vi "Multiply.vi"() -> ()   [LabVIEW 2014]
doc: "Use this template to build a VI to use as a subVI."
uses:
  <vilib>/vision/NI_Vision_Development_Module.lvlib
panel:
  out "Src":T1(plugin-control)
  out "Dst":T1(plugin-control)
  # ":: MVi Framework V1.0 ::\nAuthor:Gaoke Yang\nEmail: gaoke.yang@yahoo.com\nWeb: www.mvicontrol.com\nCopyright (C) 2015, MVI Technologies All Rights Reserved"
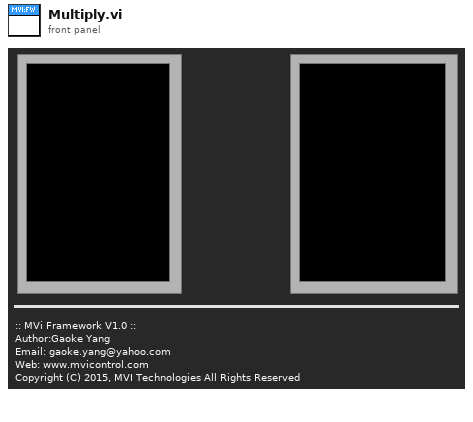
[diagram p1: front panel]
types:
  T1 = typedef "IMAQ Image.ctl" = refnum<image>
  T2 = typedef "Image Type" = u32
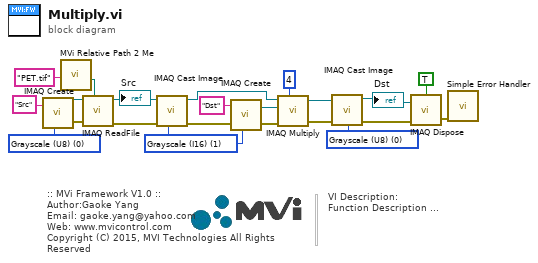
[diagram p0: block diagram]
diagram:
  w3 = T2 0 items=["Grayscale (U8)", "Grayscale (I16)", "Grayscale (SGL)", "Complex (CSG)", "RGB (U32)", "HSL (U32)", "RGB (U64)", "Grayscale (U16)"] ("Image Type")
  w2 = T2 1 items=["Grayscale (U8)", "Grayscale (I16)", "Grayscale (SGL)", "Complex (CSG)", "RGB (U32)", "HSL (U32)", "RGB (U64)", "Grayscale (U16)"] ("Image Type")
  w15 = T2 0 items=["Grayscale (U8)", "Grayscale (I16)", "Grayscale (SGL)", "Complex (CSG)", "RGB (U32)", "HSL (U32)", "RGB (U64)", "Grayscale (U16)"] ("Image Type")
  # "VI Description:\nFunction Description ..."
  # ":: MVi Framework V1.0 ::\nAuthor:Gaoke Yang\nEmail: gaoke.yang@yahoo.com\nWeb: www.mvicontrol.com\nCopyright (C) 2015, MVI Technologies All Rights Reserved"
  n1 = call "IMAQ Create"("Image Name"="Src" ("name or relative path"), "Image Type"=w15) -> ("New Image"=w16:T1, "error out"=w14:errorcluster)  [unwired: 2 in, 1 out]
  n2 = call "MVi Relative Path 2 Me.vi"("Relative Path"="PET.tif" ("name or relative path")) -> ("Appended Dir"=w18:path)  [unwired: 5 in, 1 out]
  n3 = call "IMAQ ReadFile"("File Path"=w18, "error in (no error)"=w14, "Image"=w16) -> ("error out"=w10:errorcluster, "Image Out"=w1:T1)  [unwired: 4 in, 3 out]
  "Src" <- w1
  n4 = call "IMAQ Cast Image"("Image Type"=w2, "error in (no error)"=w10, "Image Src"=w1) -> ("error out"=w9:errorcluster, "Image Dst Out"=w8:T1)  [unwired: 7 in]
  n5 = call "IMAQ Create"("Image Name"="Dst" ("name or relative path"), "Image Type"=w2, "error in (no error)"=w9) -> ("New Image"=w12:T1, "error out"=w13:errorcluster)  [unwired: 1 in, 1 out]
  n6 = call "IMAQ Multiply"("Image Src A"=w8, "Constant"=i8 4, "Image Dst"=w12, "error in (no error)"=w13) -> ("Image Dst Out"=w6:T1, "error out"=w7:errorcluster)  [unwired: 3 in]
  n7 = call "IMAQ Cast Image"("Image Type"=w3, "error in (no error)"=w7, "Image Src"=w6) -> ("error out"=w5:errorcluster, "Image Dst Out"=w4:T1)  [unwired: 7 in]
  "Dst" <- w4
  n8 = call "IMAQ Dispose"("All Images? (No)"=TRUE, "Image"=w4, "error in (no error)"=w5) -> ("error out"=w19:errorcluster)  [unwired: 3 out]
  n9 = call <vilib>:"Simple Error Handler.vi"("error in (no error)"=w19) -> ()  [unwired: 1 in, 8 out]
